vi "CreatePublicEvents.vi"(8 "error in (no error)":errorcluster, 11 "Lockin":refnum<class "Lockin.lvclass">) -> (0 "error out":errorcluster, 3 "Lockin out":refnum<class "Lockin.lvclass">)   [LabVIEW 2016, in "Lockin.lvclass"]
doc: "---------------------------------------------------------------\nJKI State Machine Objects™\nhttp://jki.net/state-machine-objects/\nCopyright (C) 2005-2015, JKI <info@jki.net>\nALL RIGHTS RESERVEDJKI State Machine Objects (SMO) 1.0.0.5\nJKI - JKI\nCopyright (c) 2016, JKI"
uses:
  Lockin.lvclass
  Typedefs/DataChanged--EventData--Cluster.ctl
  Typedefs/Data.ctl
  Lockin.lvclass/Lockin.ctl
  <vilib>/JKI/JKI SMO/SMO/SMO.lvclass
panel:
  # "For instructions on how to use the JKI State Machine Objects, examples and video tutorials, visit:\nhttp://jki.net/state-machine-objects/\n\nJKI State Machine Objects™\nhttp://jki.net/state-machine-objects/\nCopyright (C) 2005-2015, JKI <info@jki.net>\nALL RIGHTS RESERVED"
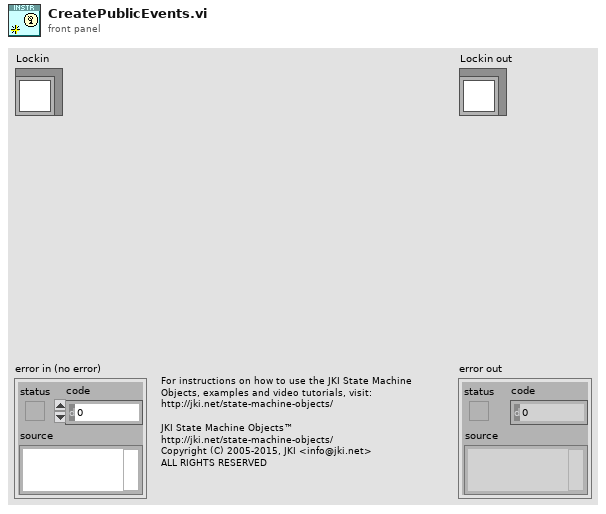
[diagram p1: front panel]
types:
  T1 = typedef "Lockin.lvclass/DataChanged--EventData--Cluster.ctl" = cluster{"Timestamp":timestamp, "Old Value":T2, "New Value":T2}
  T2 = typedef "Lockin.lvclass/Data.ctl" = string
  T3 = typedef "Lockin.lvclass/PrivateData--Ref.ctl" = refnum<data-value>
  T4 = typedef "Lockin.lvclass/PrivateData--Cluster.ctl" = cluster{"Configuration":T5, "Public Events":T6, "Protected Events":T7, "Private Events":T8, "Data":T2}
  T5 = typedef "Lockin.lvclass/Configuration--Cluster.ctl" = cluster{"Suffix":string}
  T6 = typedef "Lockin.lvclass/PublicEvents--Cluster.ctl" = cluster{"Data Changed":refnum<user-event>}
  T7 = typedef "Lockin.lvclass/ProtectedEvents--Cluster.ctl" = cluster{"API_Template":refnum<user-event>}
  T8 = typedef "Lockin.lvclass/PrivateEvents--Cluster.ctl" = cluster{"AsyncMethod":refnum<user-event>}
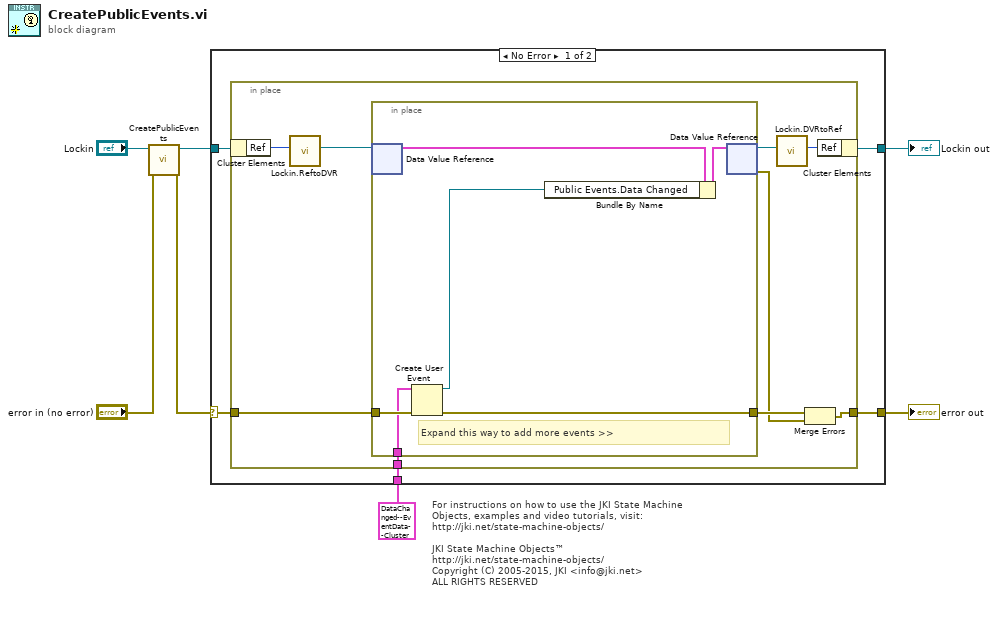
[diagram p0: block diagram]
diagram:
  # "For instructions on how to use the JKI State Machine Objects, examples and video tutorials, visit:\nhttp://jki.net/state-machine-objects/\n\nJKI State Machine Objects™\nhttp://jki.net/state-machine-objects/\nCopyright (C) 2005-2015, JKI <info@jki.net>\nALL RIGHTS RESERVED"
  n1 = call-parent "CreatePublicEvents.vi"("error in (no error)"="error in (no error)", "SMO"="Lockin") -> ("error out"=w1:errorcluster, "SMO out"=w3:refnum<class "Lockin.lvclass">)  [unwired: 8 in]
  n2 = case shown="No Error" w1 {
    selector: w1 -> [w10 w29]
    tunnel: [w9 w29] -> w6
    tunnel: [w11 w28] -> w7
    tunnel: w3 -> [w12 w28]
    tunnel: T1 {"Timestamp"=timestamp(0 s since 1904-01-01), "Old Value"="", "New Value"=""} ("Data In Event Data") -> [w8 _]
    frame No Error {
      n3 = in-place {
        in-place-border: w10 -> [w21]
        in-place-border: [w18] -> w9
        in-place-border: w8 -> [w17]
        n4 = in-place-cluster #1(w12) -> ("Ref"=w16:u32)
        n5 = call "Lockin.ReftoDVR.vi"("Ref"=w16) -> ("Ref"=w15:T3)  [unwired: 10 in]
        n6 = in-place {
          in-place-border: w21 -> [w24]
          in-place-border: [w25] -> w20
          in-place-border: w17 -> [w23]
          # "Expand this way to add more events >>"
          n7 = in-place-dvr #2(w15) -> (w26:T4)  [unwired: 1 out]
          n8 = Create User Event(user event datatype=w23, error in=w24) -> (user event=w22:refnum<user-event>, error out=w25:errorcluster)
          n9 = Bundle By Name(cluster=w26, "Public Events.Data Changed"=w22) -> (w27:T4)
          n10 = in-place-dvr #2(w27) -> (w14:T3, w19:errorcluster)
        }
        n11 = call "Lockin.DVRtoRef.vi"("Ref"=w14) -> ("Ref"=w13:u32)  [unwired: 10 in]
        n12 = Merge Errors(w20, w19) -> (w18:errorcluster)
        n13 = in-place-cluster #1("Ref"=w13) -> (w11:refnum<class "Lockin.lvclass">)
      }
    }
    frame Error {
    }
  }
  "error out" <- w6
  "Lockin out" <- w7
